vi "NISE.local.Read Sys.SessionProperties.vi"(8 "error in (no error)":errorcluster, 11 "SLSC Local in":refnum<class "SLSC Interface.lvclass">) -> (0 "error out":errorcluster, 2 "Sys.SessionProperties":refnum<k21>[](array[refnum]), 3 "SLSC Local out":refnum<class "SLSC Interface.lvclass">)   [LabVIEW 2016, in "SLSC Interface.lvclass"]
uses:
  SLSC Interface Class/SLSC Interface.lvclass
  SLSC Interface Class/NISE.Read session.vi
  <resource>/objmgr/slsc.rc
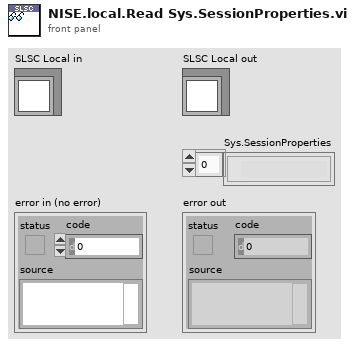
[diagram p1: front panel]
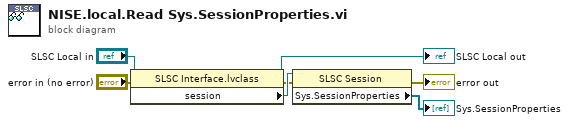
[diagram p0: block diagram]
diagram:
  n1 = property class="SLSC Interface.lvclass"(reference="SLSC Local in", error in="error in (no error)") -> (reference out=→"SLSC Local out":refnum<class "SLSC Interface.lvclass">, error out=w6:errorcluster, "session"=w7:refnum<k21>)
  n2 = property class="SLSC Session"(reference=w7, error in=w6) -> (error out=→"error out":errorcluster, "Sys.SessionProperties"=→"Sys.SessionProperties":refnum<k21>[])  [unwired: 1 out]
